vi "Verify Route.vi"(8 "error in":errorcluster, 11 "2525 in":refnum<class "2525.lvclass">) -> (0 "error out":errorcluster, 2 "Can route?":bool, 3 "2525 out":refnum<class "2525.lvclass">)   [LabVIEW 2019, in "2525.lvlib" / "2525.lvclass"]
uses:
  Library/2525.lvclass
  Library/2525.lvclass/2525.ctl
  <instrlib>/niSwitch/niSwitch.llb/niSwitch Path Capability.ctl
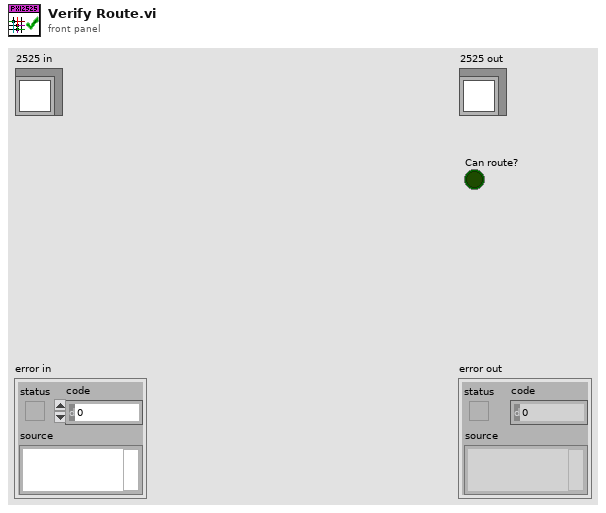
[diagram p1: front panel]
types:
  T1 = typedef "niSwitch Path Capability.ctl" = i32
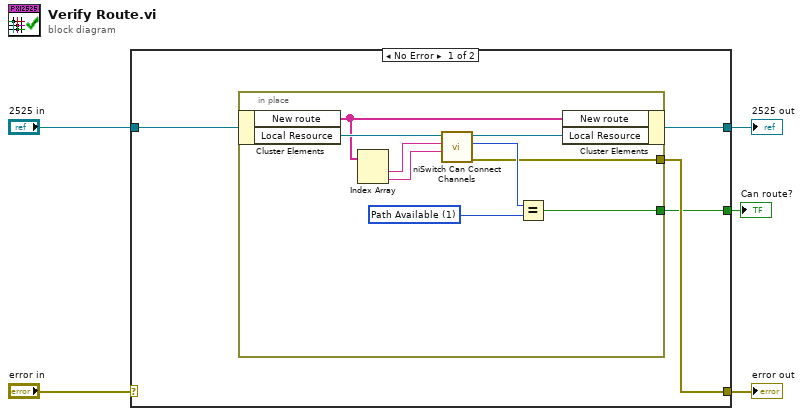
[diagram p0: block diagram]
diagram:
  n1 = case shown="No Error" "error in" {
    selector: "error in" -> [_ w20]
    tunnel: [w8 w20] -> w4
    tunnel: [w7 w19] -> w2
    tunnel: "2525 in" -> [w9 w19]
    tunnel: [w6 _] -> w1
    frame No Error {
      n2 = in-place {
        in-place-border: [w11] -> w8
        in-place-border: [w10] -> w6
        w13 = T1 1 items=["Path Available"=1, "Path Exists"=2, "Path Unsupported"=3, "Resource in Use"=4, "Source Conflict"=5, "Channel Not Available"=6] ("path capability 2")
        n3 = in-place-cluster #1(w9) -> ("New route"=w16:string[], "Local Resource"=w18:refnum<k15>)
        n4 = Index Array(array=w16) -> (element #1=w15:string, element #2=w14:string)  [unwired: 2 in]
        n5 = call <instrlib>:"niSwitch Can Connect Channels.vi"("channel 2"=w14, "channel 1"=w15, "instrument handle"=w18) -> ("error out"=w11:errorcluster, "path capability"=w12:T1, "instrument handle out"=w17:refnum<k15>)  [unwired: 6 in]
        n6 = Equal?(x=w12, y=w13) -> (x = y?=w10:bool)
        n7 = in-place-cluster #1("New route"=w16, "Local Resource"=w17) -> (w7:refnum<class "2525.lvclass">)
      }
    }
    frame Error {
    }
  }
  "error out" <- w4
  "2525 out" <- w2
  "Can route?" <- w1
